vi "Node Status to gRPC Status.vi"(2 "Node Status":T10 {"Monitor Doubles"."4" format="%#_9g"; "Monitor Doubles"."3" format="%#_9g"; "Monitor Doubles"."2" format="%#_9g"; "Monitor Doubles"."1" format="%#_9g"}) -> (4 "gRPC Status":T1)   [LabVIEW 2021, in "CIFCoreWrapper.lvlib"]
uses:
  CIFCoreWrapper.lvlib
  Common/Typedef/Plugin Status.ctl
  Common/Typedef/Plugin State.ctl
  Common/Typedef/Timing Statistics.ctl
  Common/Typedef/Timing Stats Base.ctl
  Common/Typedef/FIFO Statistics.ctl
  Common/Typedef/Simple Error.ctl
  Common/Typedef/Monitor Doubles.ctl
  Common/Typedef/Monitor U64.ctl
  Common/Typedef/Monitor I64.ctl
  CIFCorePlugin_client/RPC Messages/cif_plugincore_StatusData.ctl
  CIFCorePlugin_client/RPC Messages/cif_plugincore_StatusData_State.ctl
  CIFCorePlugin_client/RPC Messages/cif_plugincore_TimingStatistics.ctl
  CIFCorePlugin_client/RPC Messages/cif_plugincore_TimingStatsBasic.ctl
  CIFCorePlugin_client/RPC Messages/cif_plugincore_FifoStatistics.ctl
  CIFCorePlugin_client/RPC Messages/cif_plugincore_Error.ctl
  CIFCorePlugin_client/RPC Messages/cif_plugincore_MonitorDoubles.ctl
  CIFCorePlugin_client/RPC Messages/cif_plugincore_MonitorU64.ctl
  CIFCorePlugin_client/RPC Messages/cif_plugincore_MonitorI64.ctl
  CIFCorePlugin_client/CIFCorePlugin_client.lvlib
  Common/CIFCoreCommon.lvlib
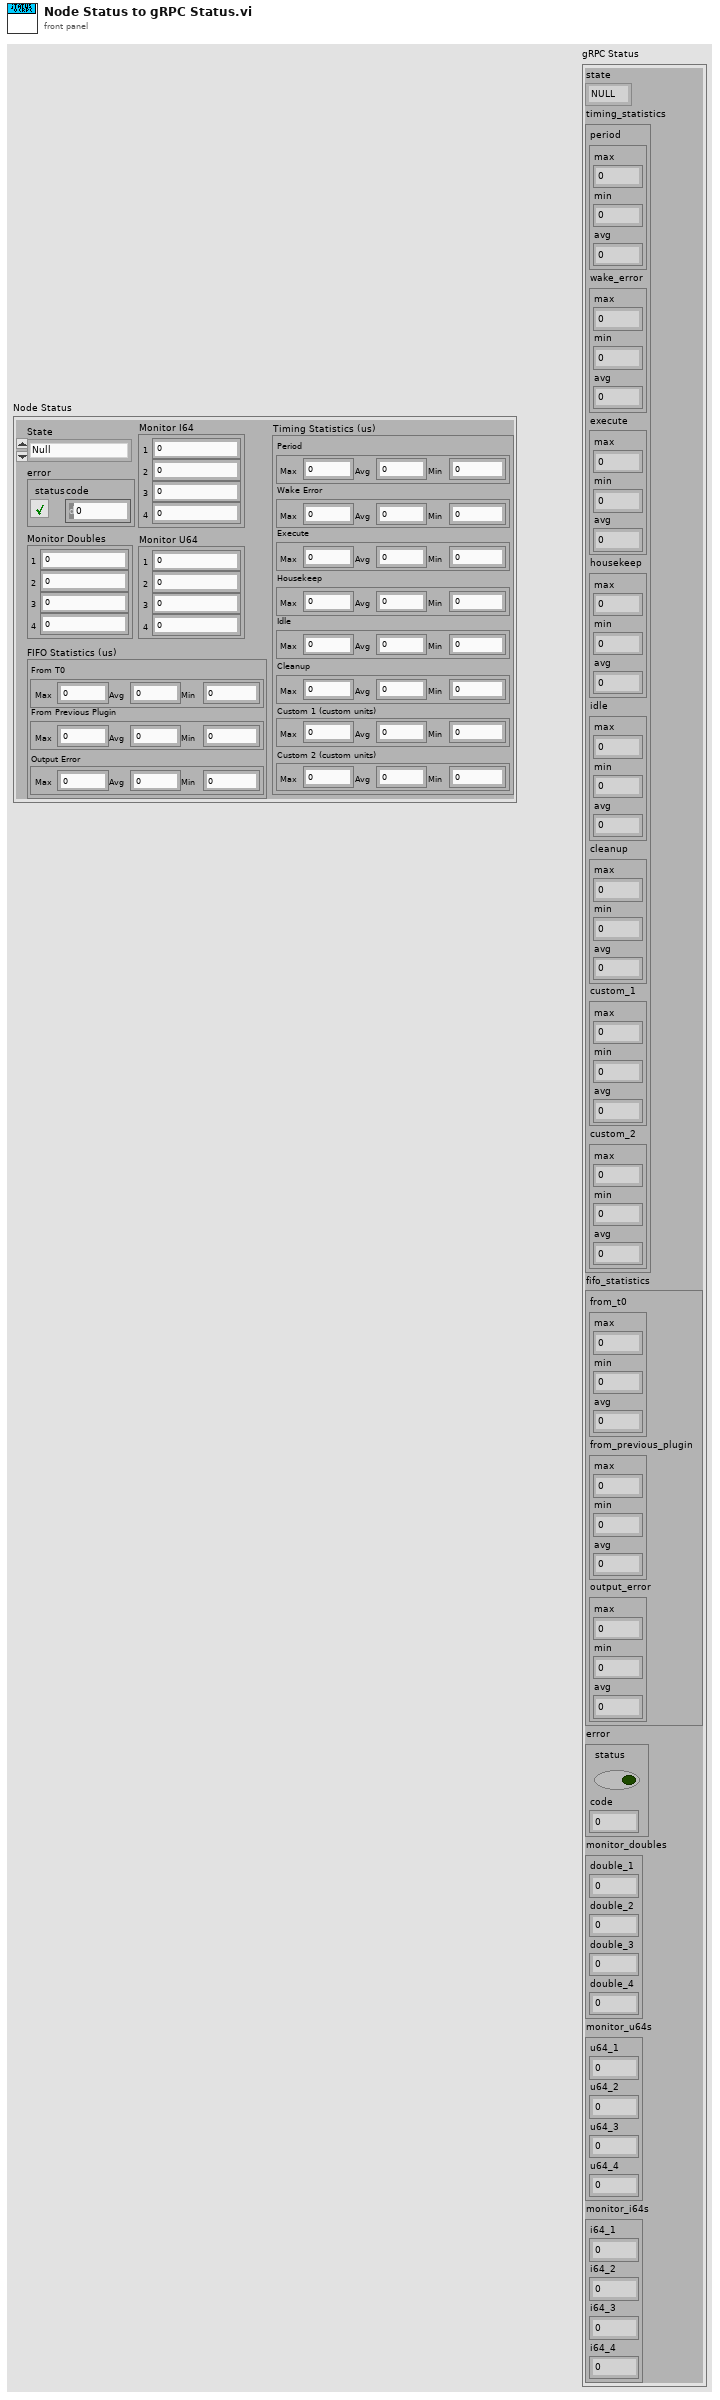
[diagram p1: front panel]
types:
  T1 = typedef "CIFCorePlugin_client.lvlib/cif_plugincore_StatusData.ctl" = cluster{"state":T2, "timing_statistics":T3, "fifo_statistics":T5, "error":T6, "monitor_doubles":T7, "monitor_u64s":T8, "monitor_i64s":T9}
  T2 = typedef "CIFCorePlugin_client.lvlib/cif_plugincore_StatusData_State.ctl" = enum32{"NULL", "CREATING", "LISTENING", "RUNNING", "CLEANINGUP", "DESTROYING"}
  T3 = typedef "CIFCorePlugin_client.lvlib/cif_plugincore_TimingStatistics.ctl" = cluster{"period":T4, "wake_error":T4, "execute":T4, "housekeep":T4, "idle":T4, "cleanup":T4, "custom_1":T4, "custom_2":T4}
  T4 = typedef "CIFCorePlugin_client.lvlib/cif_plugincore_TimingStatsBasic.ctl" = cluster{"max":i64, "min":i64, "avg":dbl}
  T5 = typedef "CIFCorePlugin_client.lvlib/cif_plugincore_FifoStatistics.ctl" = cluster{"from_t0":T4, "from_previous_plugin":T4, "output_error":T4}
  T6 = typedef "CIFCorePlugin_client.lvlib/cif_plugincore_Error.ctl" = cluster{"status":bool, "code":i32}
  T7 = typedef "CIFCorePlugin_client.lvlib/cif_plugincore_MonitorDoubles.ctl" = cluster{"double_1":dbl, "double_2":dbl, "double_3":dbl, "double_4":dbl}
  T8 = typedef "CIFCorePlugin_client.lvlib/cif_plugincore_MonitorU64.ctl" = cluster{"u64_1":u64, "u64_2":u64, "u64_3":u64, "u64_4":u64}
  T9 = typedef "CIFCorePlugin_client.lvlib/cif_plugincore_MonitorI64.ctl" = cluster{"i64_1":i64, "i64_2":i64, "i64_3":i64, "i64_4":i64}
  T10 = typedef "CIFCoreCommon.lvlib/Plugin Status.ctl" = cluster{"State":T11, "Timing Statistics (us)":T12, "FIFO Statistics (us)":T14, "error":T15, "Monitor Doubles":T16, "Monitor U64":T17, "Monitor I64":T18}
  T11 = typedef "CIFCoreCommon.lvlib/Plugin State.ctl" = enum32{"Null", "Creating", "Listening", "Running", "CleaningUp", "Destroying"}
  T12 = typedef "CIFCoreCommon.lvlib/Timing Statistics.ctl" = cluster{"Period":T13, "Wake Error":T13, "Execute":T13, "Housekeep":T13, "Idle":T13, "Cleanup":T13, "Custom 1 (custom units)":T13, "Custom 2 (custom units)":T13}
  T13 = typedef "CIFCoreCommon.lvlib/Timing Stats Base.ctl" = cluster{"Max":i64, "Avg":dbl, "Min":i64}
  T14 = typedef "CIFCoreCommon.lvlib/FIFO Statistics.ctl" = cluster{"From T0":T13, "From Previous Plugin":T13, "Output Error":T13}
  T15 = typedef "CIFCoreCommon.lvlib/Simple Error.ctl" = cluster{"status":bool, "code":i32}
  T16 = typedef "CIFCoreCommon.lvlib/Monitor Doubles.ctl" = cluster{"1":dbl, "2":dbl, "3":dbl, "4":dbl}
  T17 = typedef "CIFCoreCommon.lvlib/Monitor U64.ctl" = cluster{"1":u64, "2":u64, "3":u64, "4":u64}
  T18 = typedef "CIFCoreCommon.lvlib/Monitor I64.ctl" = cluster{"1":i64, "2":i64, "3":i64, "4":i64}
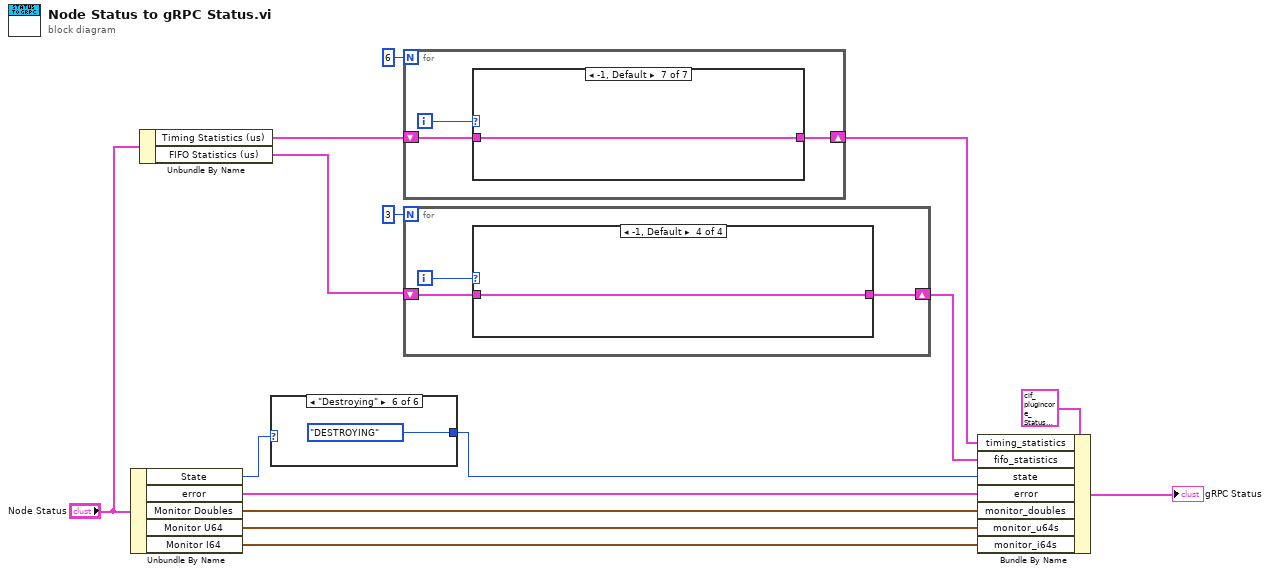
[diagram p0: block diagram]
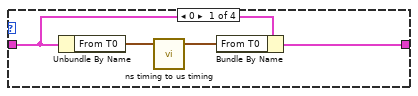
[diagram p2: hidden frame]
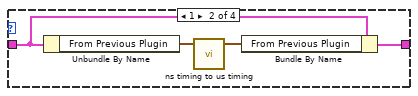
[diagram p3: hidden frame]
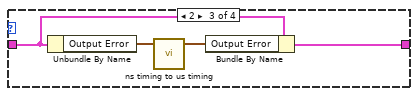
[diagram p4: hidden frame]
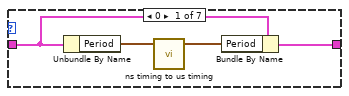
[diagram p5: hidden frame]
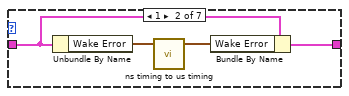
[diagram p6: hidden frame]
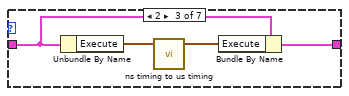
[diagram p7: hidden frame]
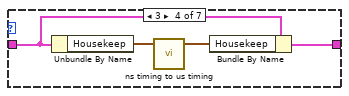
[diagram p8: hidden frame]
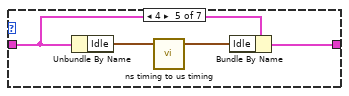
[diagram p9: hidden frame]
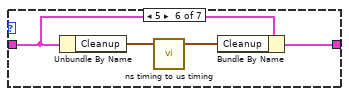
[diagram p10: hidden frame]
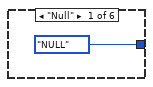
[diagram p11: hidden frame]
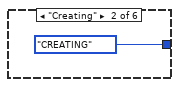
[diagram p12: hidden frame]
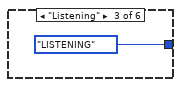
[diagram p13: hidden frame]
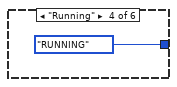
[diagram p14: hidden frame]
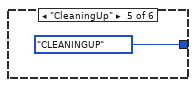
[diagram p15: hidden frame]
diagram:
  n1 = Unbundle By Name("Node Status") -> ("State"=w14:T11, "error"=w13:T15, "Monitor Doubles"=w12:T16, "Monitor U64"=w11:T17, "Monitor I64"=w10:T18)
  n2 = Unbundle By Name("Node Status") -> ("Timing Statistics (us)"=w6:T12, "FIFO Statistics (us)"=w5:T14)
  n3 = case shown="\"Destroying\"" w14 {
    tunnel: [cif_plugincore_StatusData_State."NULL" ("state") cif_plugincore_StatusData_State."CREATING" ("state") cif_plugincore_StatusData_State."LISTENING" ("state") cif_plugincore_StatusData_State."RUNNING" ("state") cif_plugincore_StatusData_State."CLEANINGUP" ("state") cif_plugincore_StatusData_State."DESTROYING" ("state")] -> w8
    frame "Null" {
    }
    frame "Creating" {
    }
    frame "Listening" {
    }
    frame "Running" {
    }
    frame "CleaningUp" {
    }
    frame "Destroying" {
    }
  }
  n4 = for {
    N: 6 -> [_]
    shift-right: [w22] -> w1
    shift-left: w6 -> [w23]
    i -> [w24]
    n5 = case shown="-1, Default" w24 {
      tunnel: w23 -> [w27 w31 w35 w39 w43 w47 w49]
      tunnel: [w25 w29 w33 w37 w41 w45 w49] -> w22
      frame 0 {
        n6 = Unbundle By Name(w27) -> ("Period"=w28:T13)
        n7 = call "ns timing to us timing.vi"("ns timing in"=w28) -> ("us timing out"=w26:T13)  [unwired: 4 in]
        n8 = Bundle By Name(cluster=w27, "Period"=w26) -> (w25:T12)
      }
      frame 1 {
        n9 = Unbundle By Name(w31) -> ("Wake Error"=w32:T13)
        n10 = call "ns timing to us timing.vi"("ns timing in"=w32) -> ("us timing out"=w30:T13)  [unwired: 4 in]
        n11 = Bundle By Name(cluster=w31, "Wake Error"=w30) -> (w29:T12)
      }
      frame 2 {
        n12 = Unbundle By Name(w35) -> ("Execute"=w36:T13)
        n13 = call "ns timing to us timing.vi"("ns timing in"=w36) -> ("us timing out"=w34:T13)  [unwired: 4 in]
        n14 = Bundle By Name(cluster=w35, "Execute"=w34) -> (w33:T12)
      }
      frame 3 {
        n15 = Unbundle By Name(w39) -> ("Housekeep"=w40:T13)
        n16 = call "ns timing to us timing.vi"("ns timing in"=w40) -> ("us timing out"=w38:T13)  [unwired: 4 in]
        n17 = Bundle By Name(cluster=w39, "Housekeep"=w38) -> (w37:T12)
      }
      frame 4 {
        n18 = Unbundle By Name(w43) -> ("Idle"=w44:T13)
        n19 = call "ns timing to us timing.vi"("ns timing in"=w44) -> ("us timing out"=w42:T13)  [unwired: 4 in]
        n20 = Bundle By Name(cluster=w43, "Idle"=w42) -> (w41:T12)
      }
      frame 5 {
        n21 = Unbundle By Name(w47) -> ("Cleanup"=w48:T13)
        n22 = call "ns timing to us timing.vi"("ns timing in"=w48) -> ("us timing out"=w46:T13)  [unwired: 4 in]
        n23 = Bundle By Name(cluster=w47, "Cleanup"=w46) -> (w45:T12)
      }
      frame -1, Default {
      }
    }
  }
  n24 = for {
    N: 3 -> [_]
    shift-right: [w50] -> w2
    shift-left: w5 -> [w51]
    i -> [w52]
    n25 = case shown="-1, Default" w52 {
      tunnel: w51 -> [w55 w57 w63 w65]
      tunnel: [w53 w58 w61 w65] -> w50
      frame 0 {
        n26 = Unbundle By Name(w55) -> ("From T0"=w56:T13)
        n27 = call "ns timing to us timing.vi"("ns timing in"=w56) -> ("us timing out"=w54:T13)  [unwired: 4 in]
        n28 = Bundle By Name(cluster=w55, "From T0"=w54) -> (w53:T14)
      }
      frame 1 {
        n29 = Unbundle By Name(w57) -> ("From Previous Plugin"=w60:T13)
        n30 = call "ns timing to us timing.vi"("ns timing in"=w60) -> ("us timing out"=w59:T13)  [unwired: 4 in]
        n31 = Bundle By Name(cluster=w57, "From Previous Plugin"=w59) -> (w58:T14)
      }
      frame 2 {
        n32 = Unbundle By Name(w63) -> ("Output Error"=w64:T13)
        n33 = call "ns timing to us timing.vi"("ns timing in"=w64) -> ("us timing out"=w62:T13)  [unwired: 4 in]
        n34 = Bundle By Name(cluster=w63, "Output Error"=w62) -> (w61:T14)
      }
      frame -1, Default {
      }
    }
  }
  n35 = Bundle By Name(cluster=T1 {"state"=enum."NULL", "timing_statistics"={"period"={"max"=0, "min"=0, "avg"=0.0}, "wake_error"={"max"=0, "min"=0, "avg"=0.0}, "execute"={"max"=0, "min"=0, "avg"=0.0}, "housekeep"={"max"=0, "min"=0, "avg"=0.0}, "idle"={"max"=0, "min"=0, "avg"=0.0}, "cleanup"={"max"=0, "min"=0, "avg"=0.0}, "custom_1"={"max"=0, "min"=0, "avg"=0.0}, "custom_2"={"max"=0, "min"=0, "avg"=0.0}}, "fifo_statistics"={"from_t0"={"max"=0, "min"=0, "avg"=0.0}, "from_previous_plugin"={"max"=0, "min"=0, "avg"=0.0}, "output_error"={"max"=0, "min"=0, "avg"=0.0}}, "error"={"status"=FALSE, "code"=0}, "monitor_doubles"={"double_1"=0.0, "double_2"=0.0, "double_3"=0.0, "double_4"=0.0}, "monitor_u64s"={"u64_1"=0, "u64_2"=0, "u64_3"=0, "u64_4"=0}, "monitor_i64s"={"i64_1"=0, "i64_2"=0, "i64_3"=0, "i64_4"=0}} ("gRPC Status"), "timing_statistics"=w1, "fifo_statistics"=w2, "state"=w8, "error"=w13, "monitor_doubles"=w12, "monitor_u64s"=w11, "monitor_i64s"=w10) -> (→"gRPC Status":T1)
